vi "CAL_PRESSURE_TRANSDUCER.vi"(7 "Array in":refnum<k24>[](array[refnum]), 8 "error in (no error)":errorcluster, 9 "Descriptions":string[](array[string]), 10 "Sensor Cluster":T1, 11 "pressure_slope_IN":dbl=51.35 format="%.2f") -> (0 "error out":errorcluster, 3 "pressure_slope_OUT":dbl=51.35 format="%.2f", 5 "Array out":refnum<k24>[](array[refnum]))   [LabVIEW 2016]
uses:
  Waterloo DAQ/controls/MCC DAQ Readings.ctl
  C:/Program Files (x86)/National Instruments/LabVIEW 2016/vi.lib/ULx/ULx_LV.dll
  ad interface/Global_SIM_switch.vi
  Kpro Globals.vi
panel:
  out "ok":bool
  out "zero":bool
  out "Pressure":dbl format="%.2f"
  in  "ok":bool
  in  "zero":bool
  # "PRESSURE TRANSDUCER CALIBRATION"
  # "(step 1)"
  # "Fill graduated cylinder to 750 mL water.\nSubmerge Kpro effluent and start flow.\nStop flow at 800 mL of water (1 foot).\nAllow pressure to equilibrate and press zero."
  # "(step 2)"
  # "Hold Kpro effluent facing up and 5' above the floor.\nTurn Kpro flow on briefly to fill the Kpro line.\nTurn Kpro flow off again.\nPress OK when pressure has equilibrated"
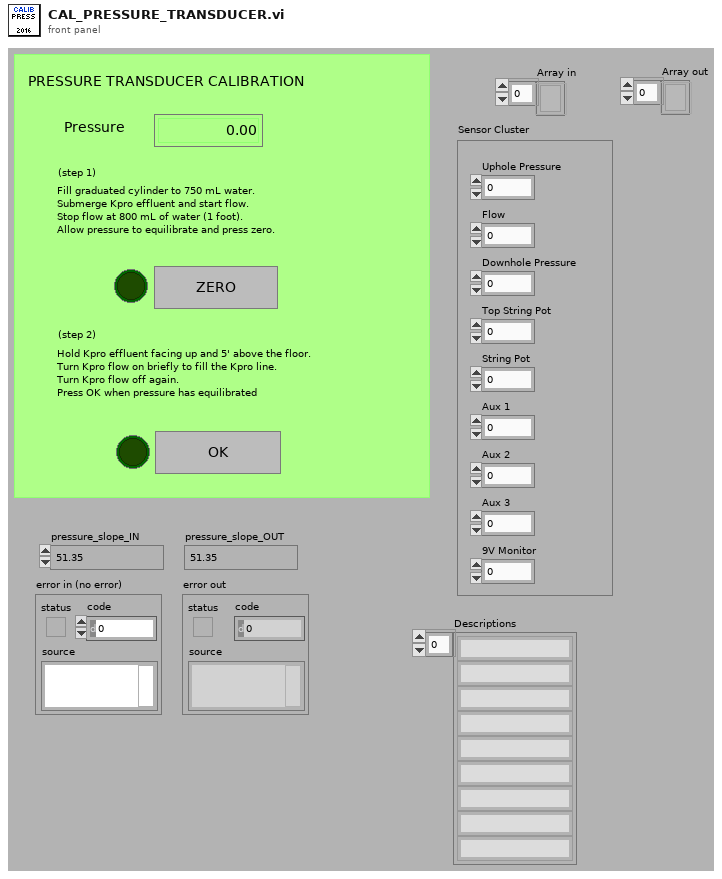
[diagram p1: front panel]
types:
  T1 = typedef "MCC DAQ Readings.ctl" = cluster{"Uphole Pressure":dbl, "Flow":dbl, "Downhole Pressure":dbl, "Top String Pot":dbl, "String Pot":dbl, "Aux 1":dbl, "Aux 2":dbl, "Aux 3":dbl, "9V Monitor":dbl}
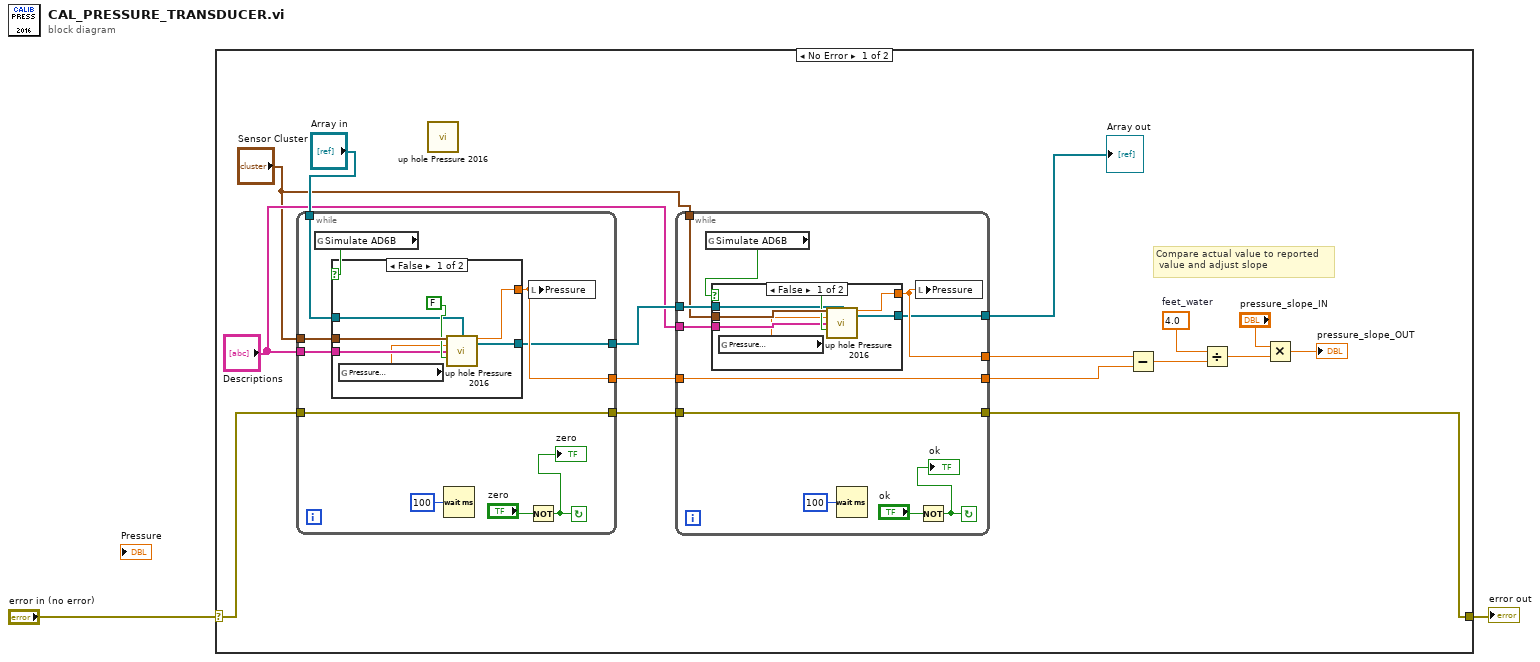
[diagram p0: block diagram]
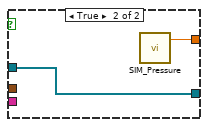
[diagram p2: hidden frame]
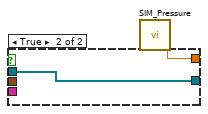
[diagram p3: hidden frame]
diagram:
  n1 = case shown="No Error" "error in (no error)" {
    selector: "error in (no error)" -> [w18 w58]
    tunnel: [w16 w58] -> w2
    frame No Error {
      w14 = 4.0  # feet_water
      # "Compare actual value to reported\n value and adjust slope"
      n2 = while {
        tunnel: [w25] -> w8
        tunnel: [w27] -> w17
        tunnel: w18 -> [w27]
        tunnel: "Sensor Cluster" -> [w22]
        tunnel: "Array in" -> [w21]
        tunnel: [w20] -> w6
        tunnel: "Descriptions" -> [w19]
        stop <- w23 continue-if-true
        n3 = global read "Global_SIM_switch.vi" "Simulate AD6B"() -> (w26:bool)
        n4 = case shown="False" w26 {
          tunnel: [w33 w37] -> w25
          tunnel: w22 -> [w35 _]
          tunnel: w21 -> [w32 w36]
          tunnel: [w31 w36] -> w20
          tunnel: w19 -> [w30 _]
          frame False {
            n5 = global read "Kpro Globals.vi" "Pressure \nSlope"() -> (w29:dbl)
            n6 = call "up hole Pressure 2016.vi"("Sensor Cluster"=w35, "Array in"=w32, "Pressure \nSlope"=w29, "Descriptions"=w30, "Zero Pressure\n(F = leave as is)"=FALSE ("Zero Pressure\n(F = leave as is)")) -> ("Array out"=w31:refnum<k24>[], "Uphole Pressure"=w33:dbl)  [unwired: 9 in]
          }
          frame True {
            n7 = call "SIM_Pressure.vi"() -> ("Pressure"=w37:dbl)  [unwired: 11 in]
          }
        }
        n8 = Wait (ms)(milliseconds to wait=u32 100) -> ()  [unwired: 1 out]
        n9 = Not(x="zero") -> (.not. x?=w23:bool)
        "zero" <- w23
        n10 = local write "Pressure"(w25) -> ()
      }
      n11 = call "up hole Pressure 2016.vi"() -> ()  [unwired: 14 in, 2 out]
      n12 = while {
        tunnel: w8 -> [w46]
        tunnel: [w43] -> w11
        tunnel: [w46] -> w15
        tunnel: w17 -> [w47]
        tunnel: [w47] -> w16
        tunnel: w6 -> [w41]
        tunnel: [w40] -> w5
        tunnel: "Descriptions" -> [w39]
        tunnel: "Sensor Cluster" -> [w38]
        stop <- w44 continue-if-true
        n13 = global read "Global_SIM_switch.vi" "Simulate AD6B"() -> (w42:bool)
        n14 = case shown="False" w42 {
          tunnel: [w53 w57] -> w43
          tunnel: w38 -> [w55 _]
          tunnel: w41 -> [w52 w56]
          tunnel: [w51 w56] -> w40
          tunnel: w39 -> [w50 _]
          frame False {
            n15 = global read "Kpro Globals.vi" "Pressure \nSlope"() -> (w49:dbl)
            n16 = call "up hole Pressure 2016.vi"("Sensor Cluster"=w55, "Array in"=w52, "Pressure \nSlope"=w49, "Descriptions"=w50, "Zero Pressure\n(F = leave as is)"=FALSE ("Zero Pressure\n(F = leave as is)")) -> ("Array out"=w51:refnum<k24>[], "Uphole Pressure"=w53:dbl)  [unwired: 9 in]
          }
          frame True {
            n17 = call "SIM_Pressure.vi"() -> ("Pressure"=w57:dbl)  [unwired: 11 in]
          }
        }
        n18 = Wait (ms)(milliseconds to wait=u32 100) -> ()  [unwired: 1 out]
        n19 = local write "Pressure"(w43) -> ()
        n20 = Not(x="ok") -> (.not. x?=w44:bool)
        "ok" <- w44
      }
      "Array out" <- w5
      n21 = Subtract(x=w11, y=w15) -> (x-y=w10:dbl)
      n22 = Divide(x=w14, y=w10) -> (x/y=w9:dbl)
      n23 = Multiply(x="pressure_slope_IN", y=w9) -> (x*y=→"pressure_slope_OUT":dbl)
    }
    frame Error {
    }
  }
  "error out" <- w2
